vi "DB Update Array Data(Feedback).vi"(6 "index":i32, 7 "Data":string[](array[string]), 8 "error in (no error)":errorcluster caption="错误输入（无错误）", 9 "columns":string[](array[string]), 10 "table name":string, 11 "Connncet State":T1) -> (0 "error out":errorcluster caption="错误输出", 1 "布尔":bool, 3 "Connncet State out":T1)   [LabVIEW 2014]
uses:
  Ctr/Constr.ctl
  <vilib>/addons/database/Connection.llb/Conn ObjectReference.ctl
  <vilib>/addons/database/NI_Database_API.lvlib
  Ctr/Conneect State.ctl
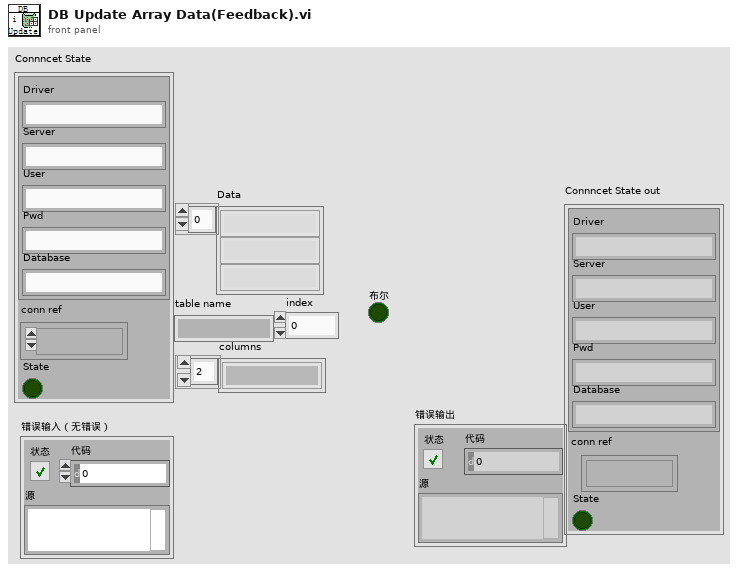
[diagram p1: front panel]
types:
  T1 = typedef "Conneect State.ctl" = cluster{"Constr":T2, "conn ref":T3, "State":bool}
  T2 = typedef "Constr.ctl" = cluster{"Driver":string, "Server":string, "User":string, "Pwd":string, "Database":string}
  T3 = typedef "NI_Database_API.lvlib/Conn ObjectReference.ctl" = refnum<k1>
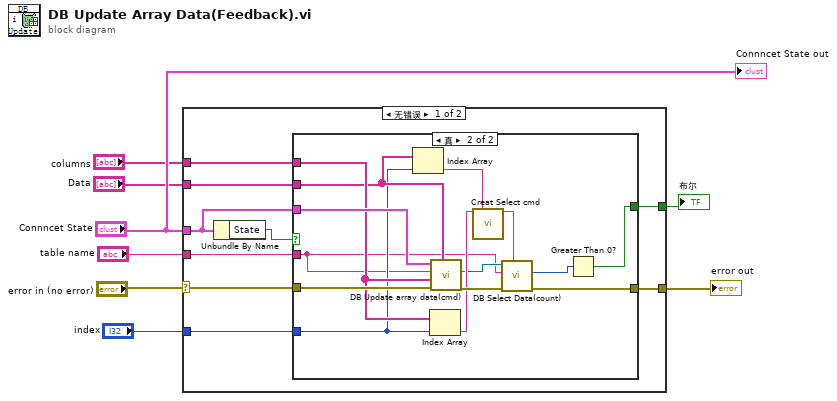
[diagram p0: block diagram]
diagram:
  n1 = case shown="无错误" "error in (no error)" {
    selector: "error in (no error)" -> [w17 w33]
    tunnel: "Connncet State" -> [w13 _]
    tunnel: [w15 w33] -> w2
    tunnel: [w14 _] -> w1
    tunnel: "Data" -> [w12 _]
    tunnel: "table name" -> [w11 _]
    tunnel: "columns" -> [w10 _]
    tunnel: "index" -> [w9 _]
    frame No Error {
      n2 = Unbundle By Name(w13) -> ("State"=w16:bool)
      n3 = case shown="真" w16 {
        tunnel: w17 -> [w18 w29]
        tunnel: [w18 w31] -> w15
        tunnel: [_ w20] -> w14
        tunnel: w13 -> [_ w30]
        tunnel: w12 -> [_ w26]
        tunnel: w11 -> [_ w22]
        tunnel: w10 -> [_ w28]
        tunnel: w9 -> [_ w25]
        frame False {
        }
        frame True {
          n4 = Index Array(array=w26, index=w25) -> (element=w24:string)
          n5 = Index Array(array=w28, index=w25) -> (element=w27:string)
          n6 = call "DB Update array data(cmd).vi"("Data"=w26, "error in (no error)"=w29, "columns"=w28, "table name"=w22, "Connncet State"=w30) -> ("error out"=w32:errorcluster, "connection reference"=w23:T3)  [unwired: 4 in, 1 out]
          n7 = call "Creat Select cmd.vi"("Col"=w27, "Code"=w24) -> ("Str"=w19:string)  [unwired: 12 in, 1 out]
          n8 = call "DB Select Data(count).vi"("condition"=w19, "error in (no error)"=w32, "table"=w22, "connection reference"=w23) -> ("error out"=w31:errorcluster, "Count"=w21:i32)  [unwired: 5 in, 1 out]
          n9 = Greater Than 0?(x=w21) -> (x > 0?=w20:bool)
        }
      }
    }
    frame Error {
    }
  }
  "error out" <- w2
  "布尔" <- w1
  "Connncet State out" <- "Connncet State"
